vi "LED WIP.vi"() -> ()   [LabVIEW 2018]
panel:
  out "Colors [4]":cluster{u32, u32}[](array[cluster])
  out "Boolean Round":bool
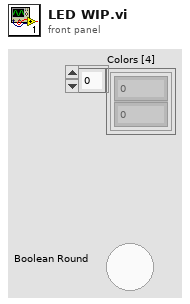
[diagram p1: front panel]
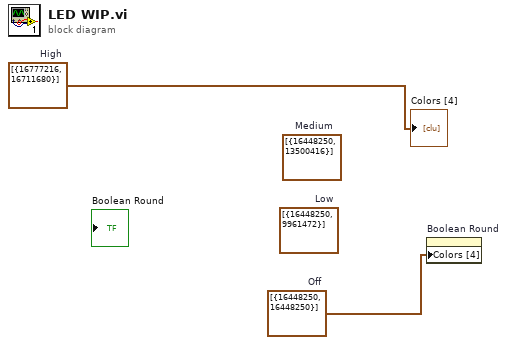
[diagram p0: block diagram]
diagram:
  w1 = cluster{u32, u32}[] [{16448250, 16448250}]  # Off
  (unwired) cluster{u32, u32}[] [{16448250, 9961472}]  # Low
  (unwired) cluster{u32, u32}[] [{16448250, 13500416}]  # Medium
  w2 = cluster{u32, u32}[] [{16777216, 16711680}]  # High
  n1 = property on="Boolean Round" class="Bool (strict)"("Colors [4]"=w1) -> ()  [unwired: 2 in, 2 out]
  "Colors [4]" <- w2
